vi "Insert_Array.vi"() -> ()   [LabVIEW 2020]
panel:
  in  "New Element":dbl
  out "Result":dbl[](array[numeric])
  in  "List1":dbl[](array[numeric])
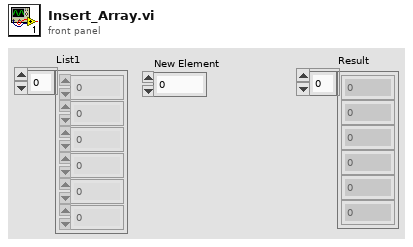
[diagram p1: front panel]
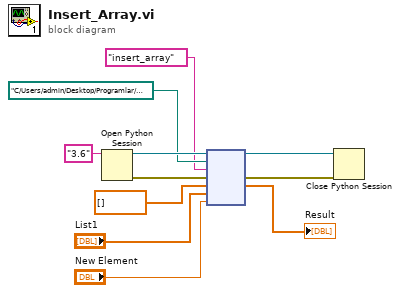
[diagram p0: block diagram]
diagram:
  n1 = Open Python Session(python version="3.6" ("Python version")) -> (session out=w11:refnum<k35>, error out=w10:errorcluster)  [unwired: 2 in]
  n2 = node(w11, path "C:/Users/admin/Desktop/Programlar/Python/Basic Examples/Pyton Code/Array_List.py" ("module path"), "insert_array" ("function name"), w10, dbl[] [], "List1", "New Element") -> (w9:refnum<k35>, w8:errorcluster, →"Result":dbl[])  [unwired: 2 in, 2 out]
  n3 = Close Python Session(session in=w9, error in=w8) -> ()  [unwired: 1 out]
